vi "APT Control.vi"() -> ()   [LabVIEW 2015]
panel:
  in  "MG17Motor 5":refnum<k7>(container)
  in  "MG17Motor 4":refnum<k7>(container)
  in  "MG17Motor 3":refnum<k7>(container)
  in  "MG17Motor 2":refnum<k7>(container)
  in  "选项卡控件":enum32{"APT Controller", "Parameters"}(tab)
  in  "STOP Device":bool
  in  "Absolute 5":dbl
  in  "Absolute 4":dbl=1.0
  in  "Absolute 3":dbl
  in  "Absolute 2":dbl
  in  "Absolute 1":dbl
  in  "Stop":bool=TRUE
  in  "Home 1":bool
  in  "Rel. Pos 1":dbl=0.01 min=-10.0 max=360.0 format="%.2f"
  out "Display 1":dbl(knob) scale=0.0..50.0
  out "Initial 1":bool=TRUE
  in  "HWSerialNum 1":i32=90868400
  in  "1 Down":bool
  in  "1 Up":bool
  in  "HWSerialNum 2":i32=90868399
  out "Initial 2":bool=TRUE
  out "Display 2":dbl(knob) scale=0.0..25.0
  in  "2 Up":bool
  in  "2 Down":bool
  in  "HWSerialNum 3":i32=90843970
  out "Initial 3":bool=TRUE
  out "Display 3":dbl(knob)=0.9999828934669495 scale=0.0..25.0
  in  "3 Up":bool
  in  "3 Down":bool
  in  "Rel. Pos 3":dbl=0.01 min=-10.0 max=360.0 format="%.2f"
  in  "HWSerialNum 4":i32=90843969
  out "Initial 4":bool=TRUE
  out "Display 4":dbl(knob)=1.0 scale=0.0..50.0
  in  "4 Up":bool
  in  "4 Down":bool
  in  "Rel. Pos 4":dbl=0.1 min=-10.0 max=360.0 format="%.2f"
  in  "HWSerialNum 5":i32=90843968
  out "Initial 5":bool=TRUE
  out "Display 5":dbl(knob)=1.7000000476837158 scale=0.0..50.0
  in  "5 Up":bool
  in  "5 Down":bool
  in  "Rel. Pos 5":dbl=1.0 min=-10.0 max=360.0 format="%.2f"
  in  "Home 2":bool
  in  "Home 3":bool
  in  "Home 4":bool
  in  "Home 5":bool
  in  "Rel. Pos 2":dbl=0.01 min=-10.0 max=360.0 format="%.2f"
  in  "MG17Motor 1":refnum<k7>(container)
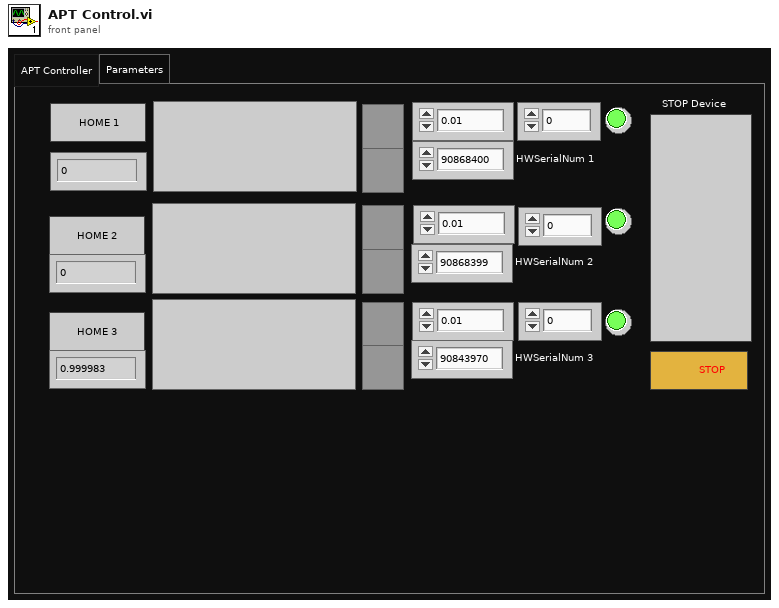
[diagram p1: front panel]
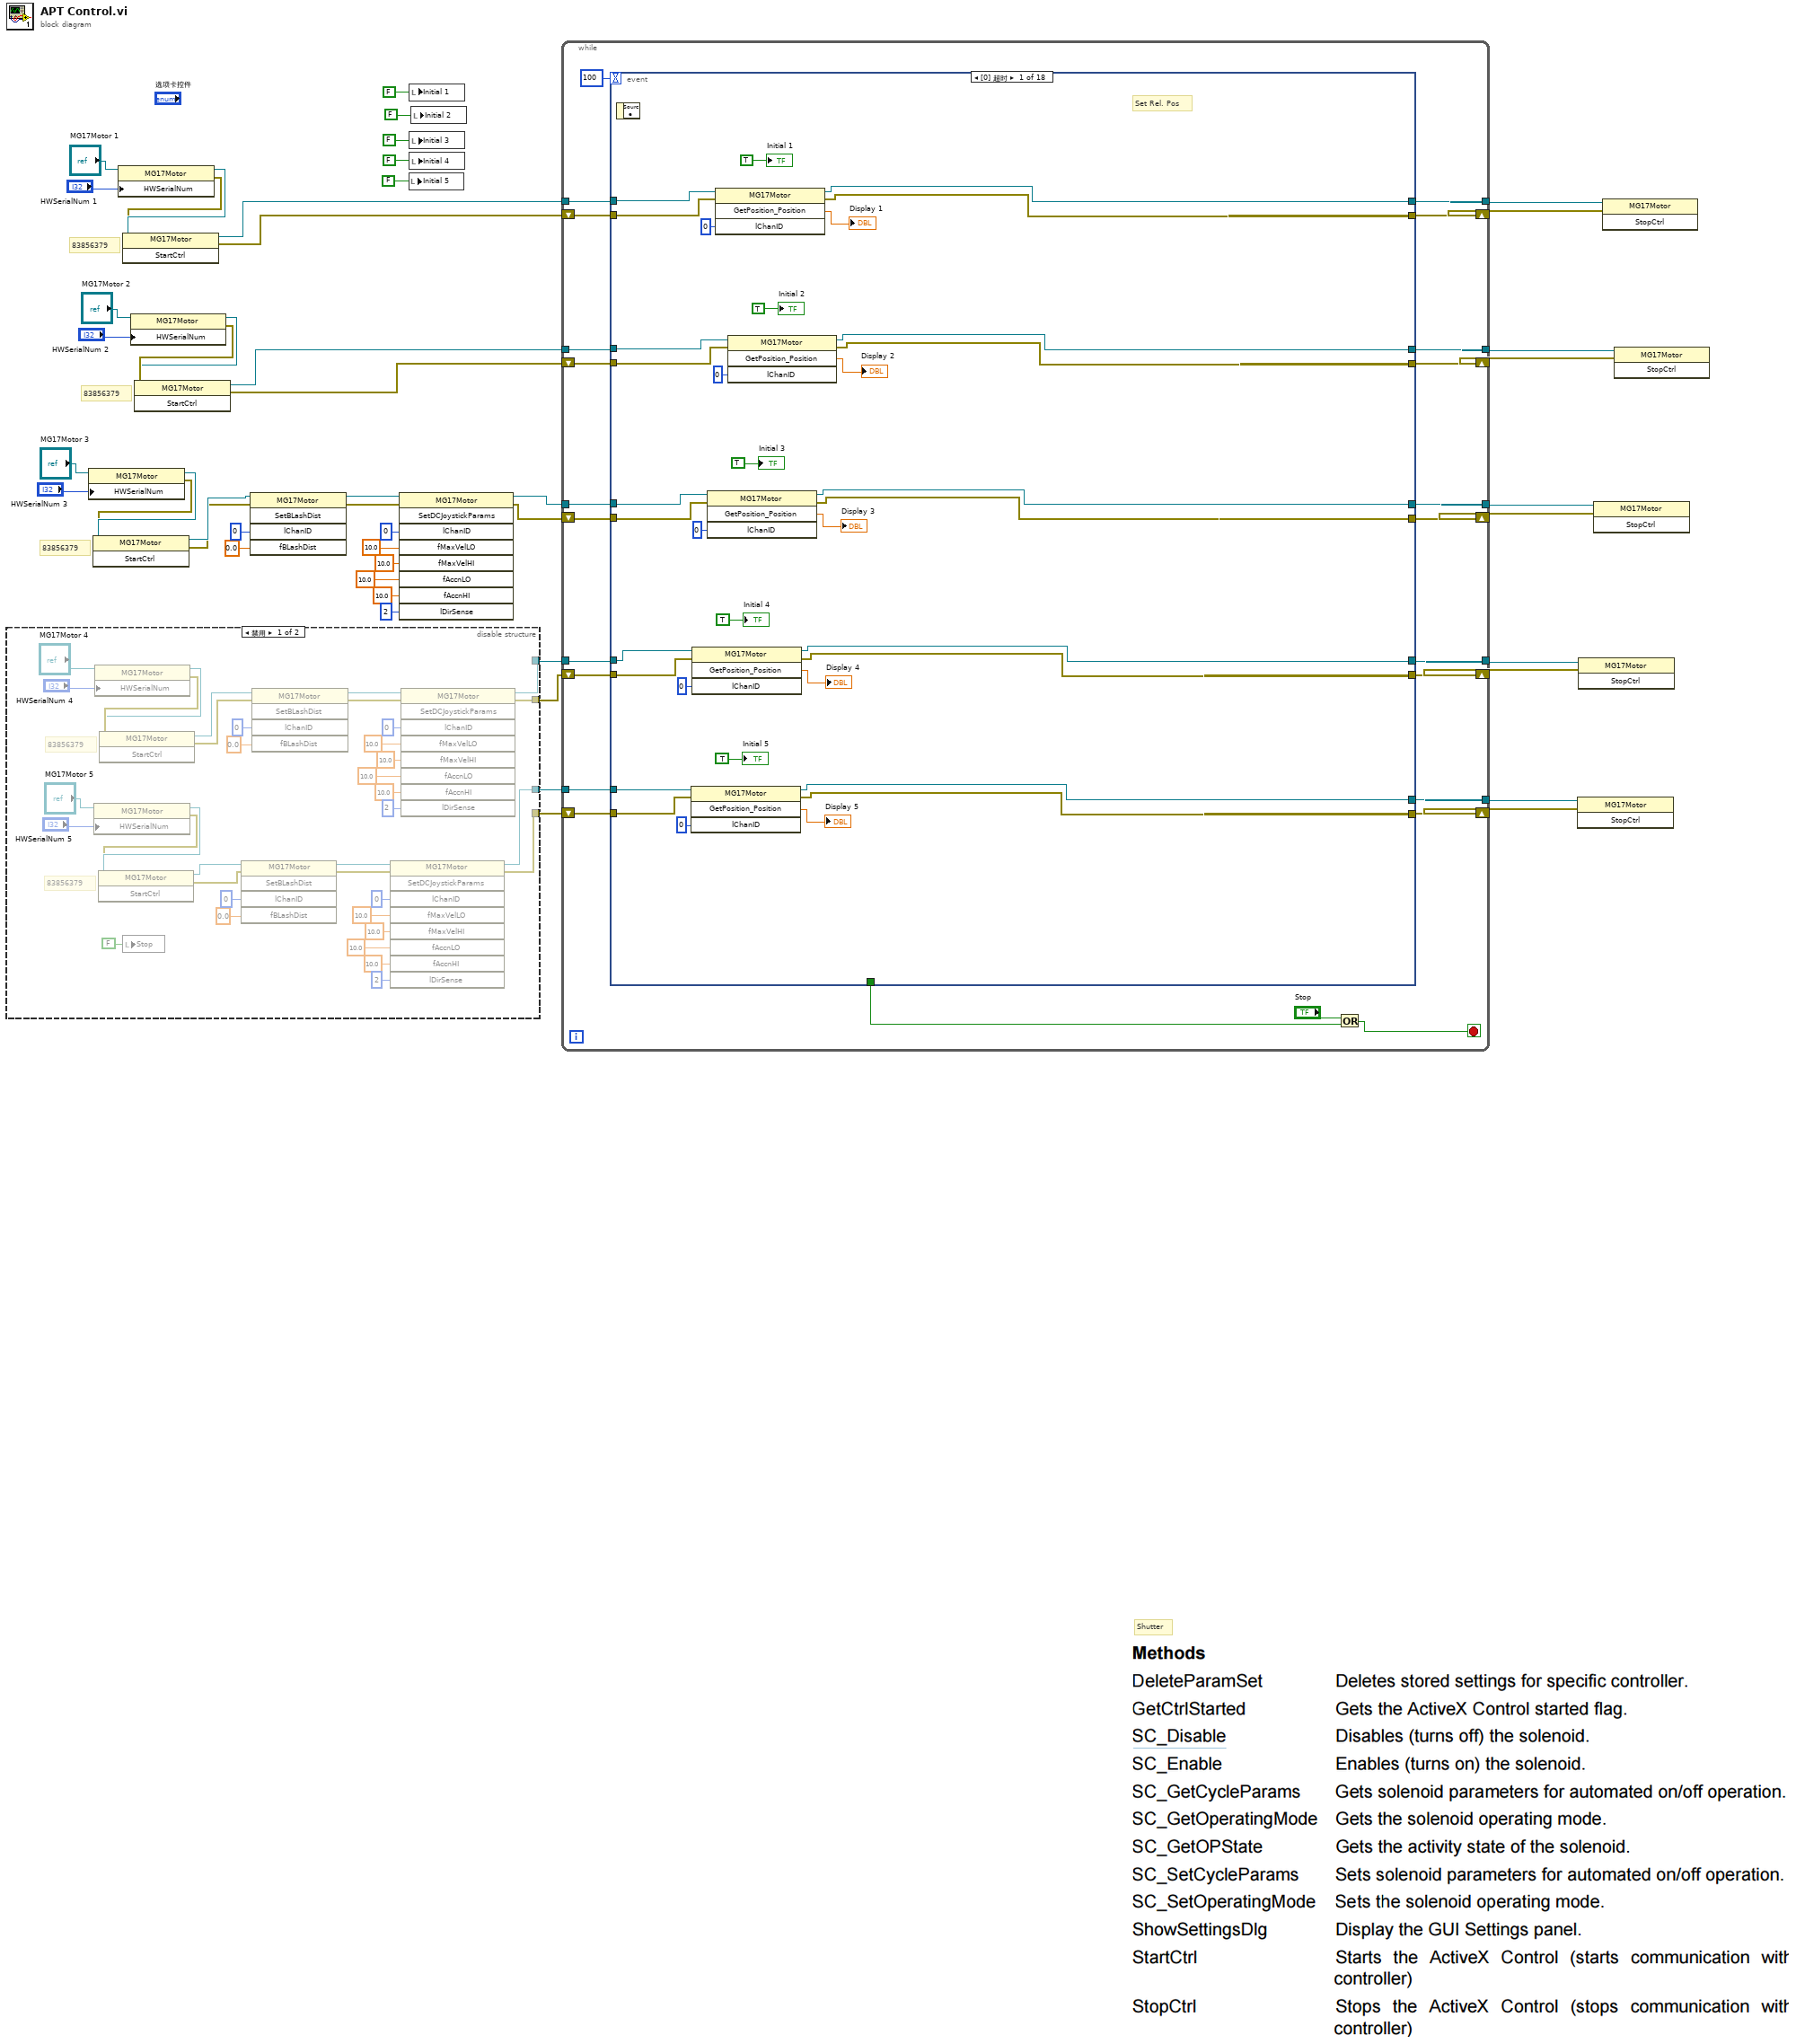
[diagram p0: block diagram]
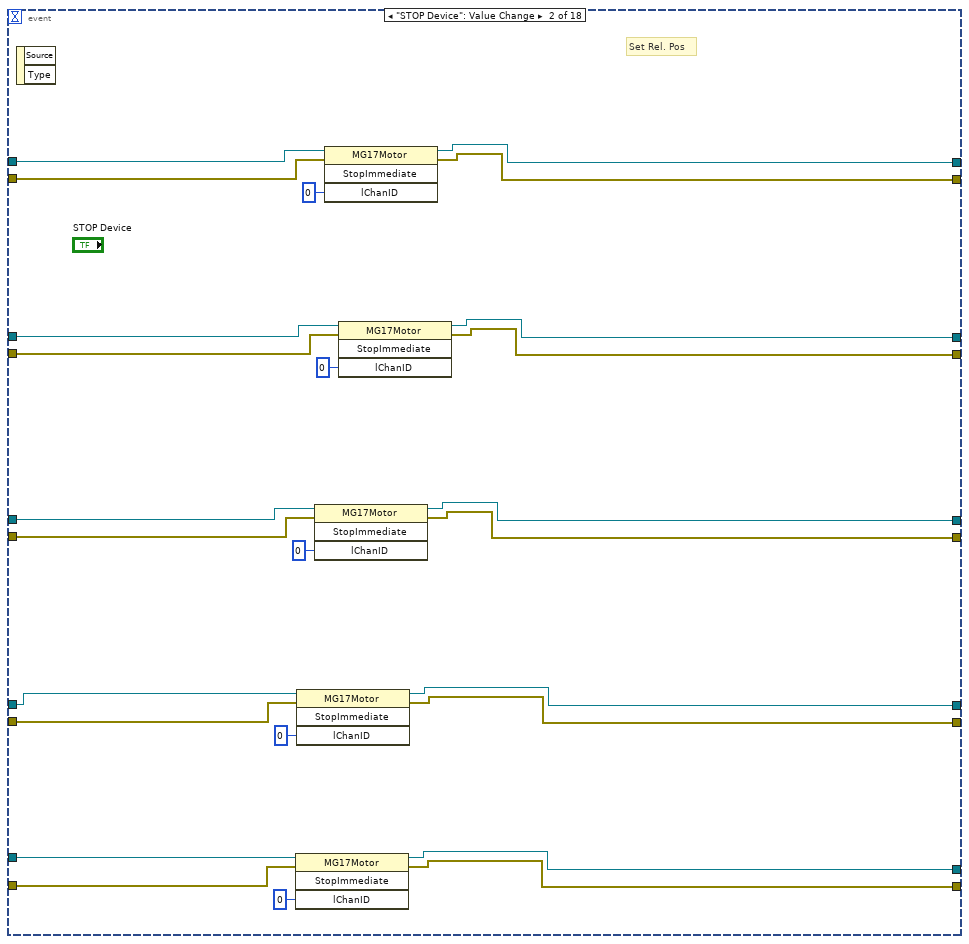
[diagram p3: hidden frame]
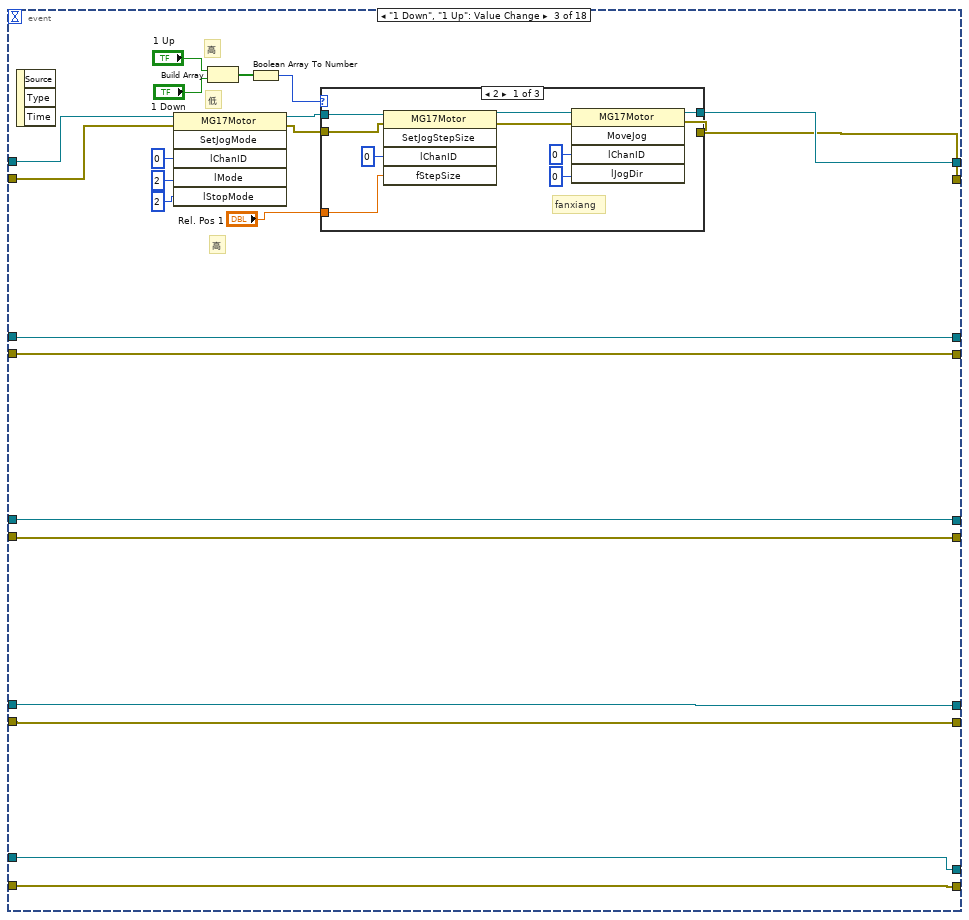
[diagram p4: hidden frame]
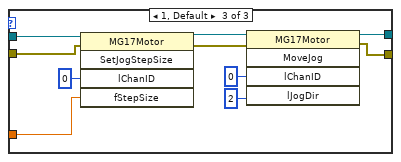
[diagram p6: hidden frame]
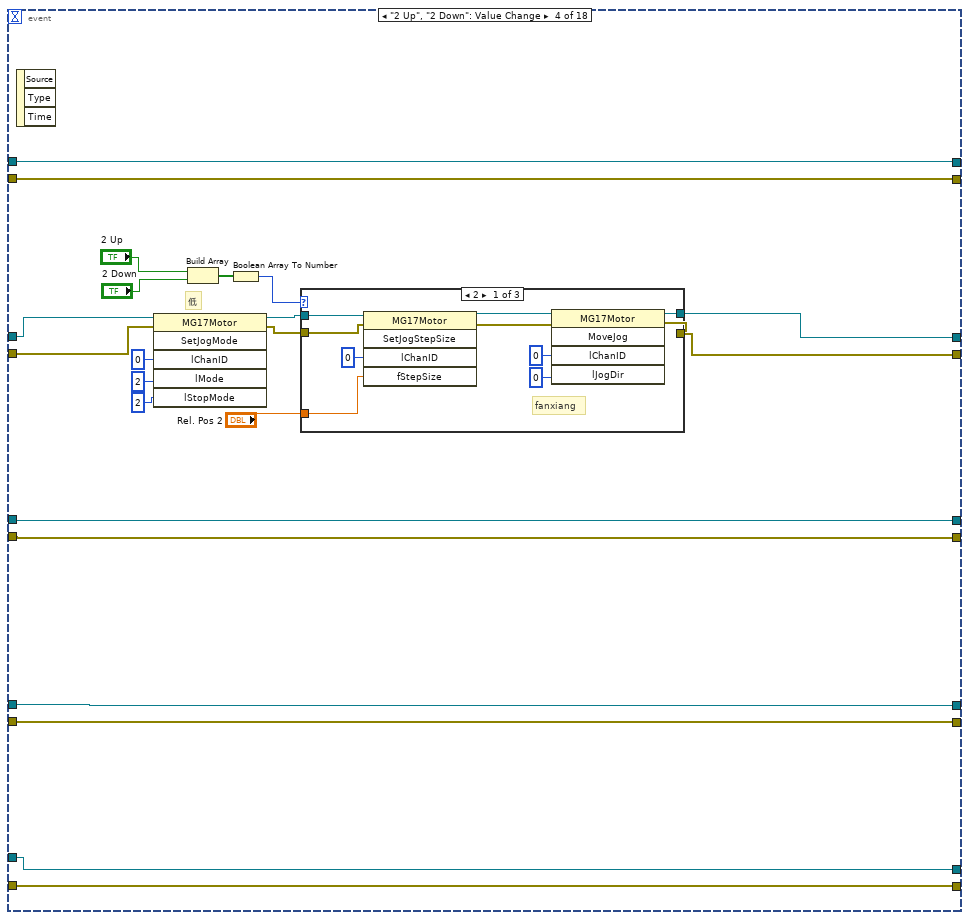
[diagram p7: hidden frame]
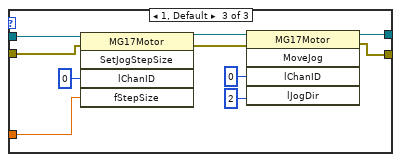
[diagram p9: hidden frame]
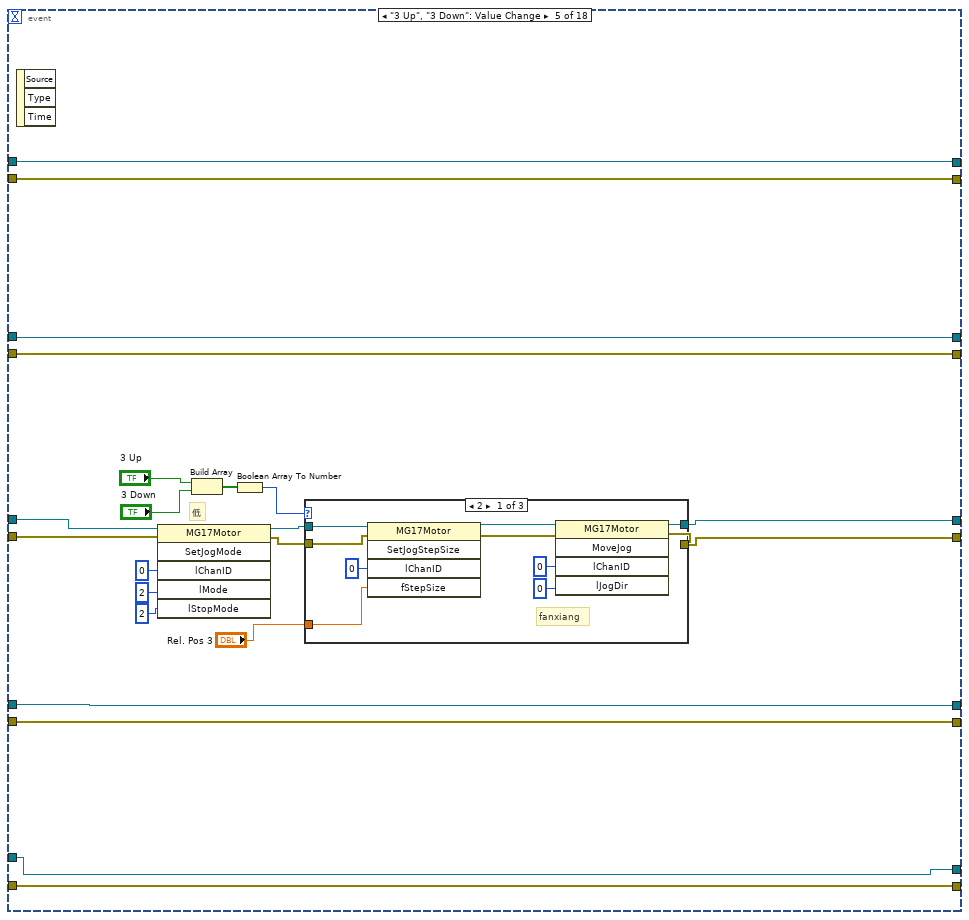
[diagram p10: hidden frame]
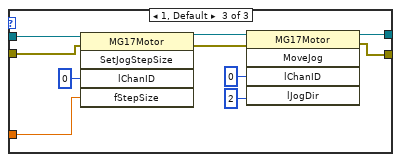
[diagram p12: hidden frame]
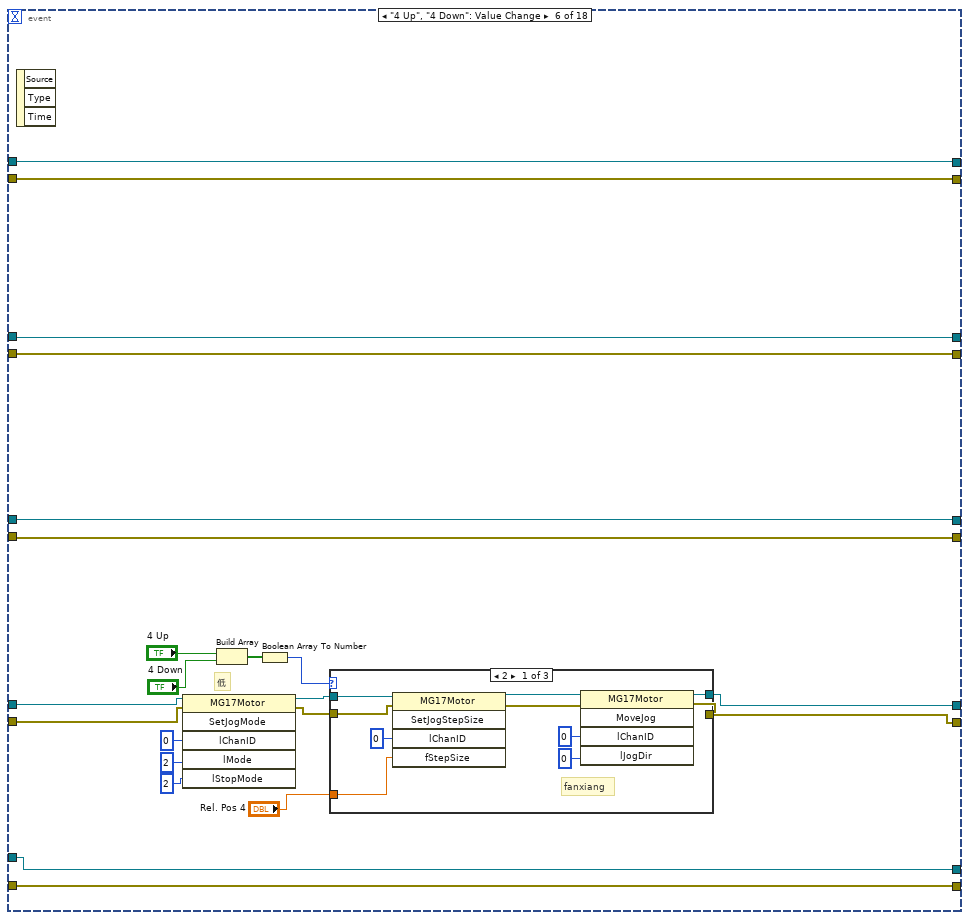
[diagram p13: hidden frame]
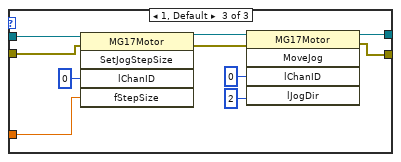
[diagram p15: hidden frame]
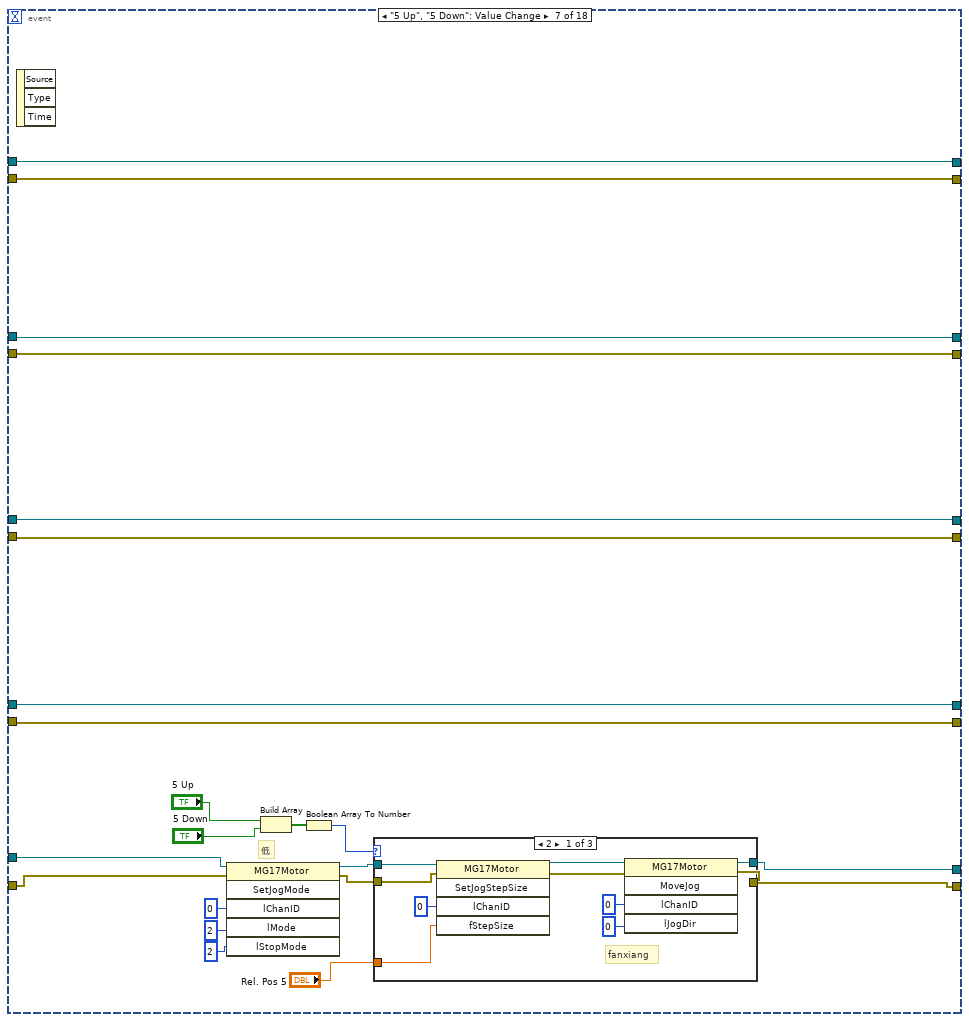
[diagram p16: hidden frame]
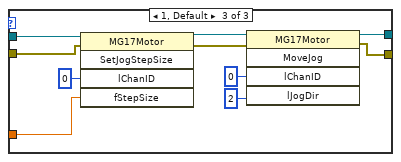
[diagram p18: hidden frame]
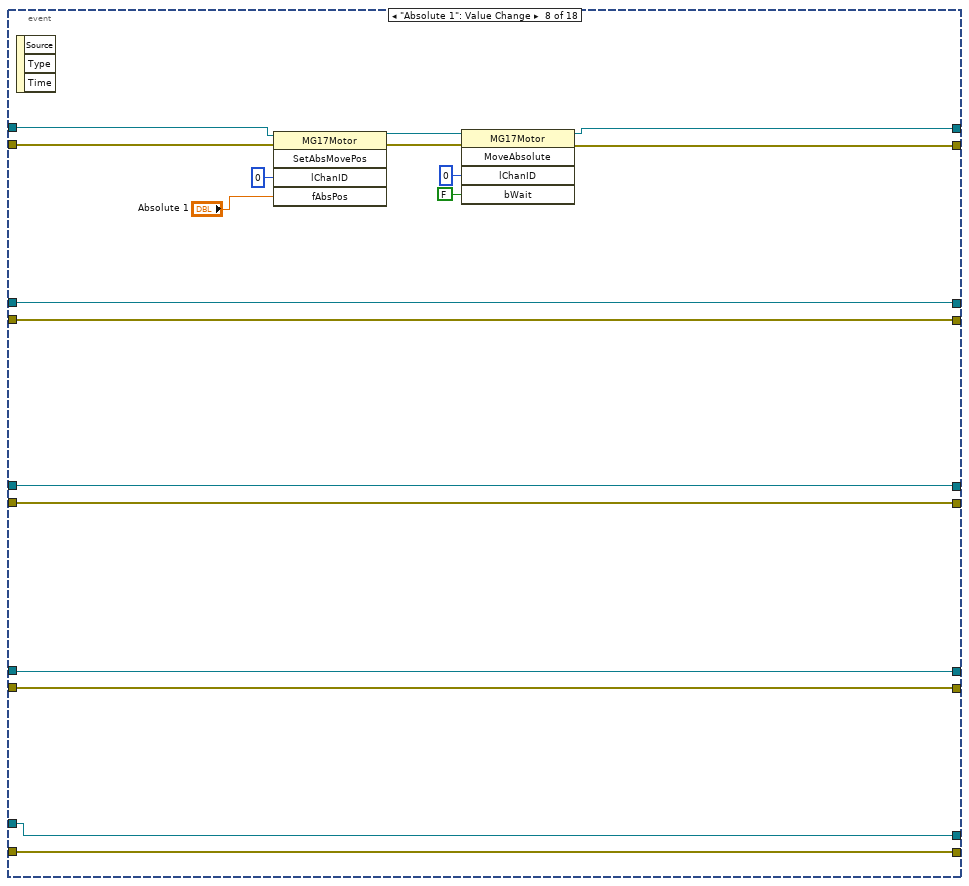
[diagram p19: hidden frame]
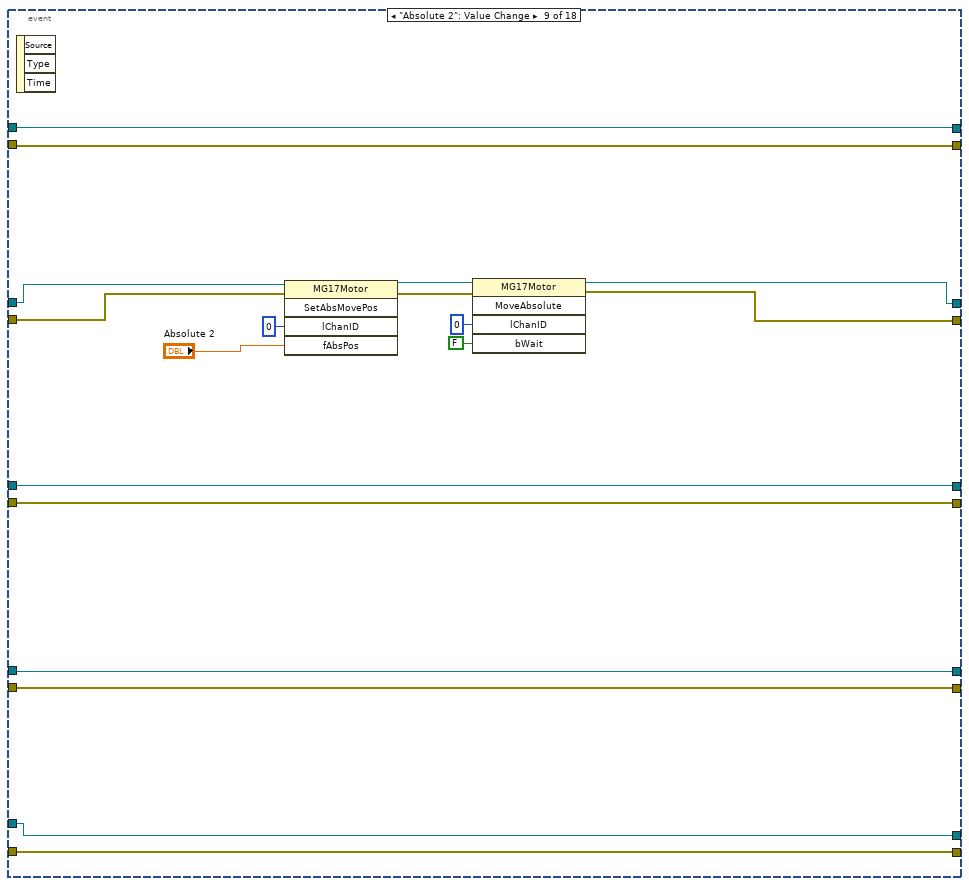
[diagram p20: hidden frame]
diagram:
  # "83856379"
  # "83856379"
  # "83856379"
  # "Shutter"
  n1 = disable-structure shown="禁用" {
    disable-tunnel: [w57 _] -> w18
    disable-tunnel: [w56 _] -> w17
    disable-tunnel: [w55 _] -> w16
    disable-tunnel: [w54 _] -> w15
    frame Disabled {
      # "83856379"
      # "83856379"
      n2 = property class="MG17Motor"(reference="MG17Motor 5", "HWSerialNum"="HWSerialNum 5") -> (reference out=w81:refnum<k7>, error out=w80:errorcluster)  [unwired: 1 in]
      n3 = property class="MG17Motor"(reference="MG17Motor 4", "HWSerialNum"="HWSerialNum 4") -> (reference out=w84:refnum<k7>, error out=w85:errorcluster)  [unwired: 1 in]
      n4 = invoke class="MG17Motor" method="StartCtrl"(reference=w81, error in=w80) -> (reference out=w53:refnum<k7>, error out=w52:errorcluster)  [unwired: 1 in, 1 out]
      n5 = invoke class="MG17Motor" method="StartCtrl"(reference=w84, error in=w85) -> (reference out=w51:refnum<k7>, error out=w50:errorcluster)  [unwired: 1 in, 1 out]
      n6 = local write "Stop"(FALSE ("Stop")) -> ()
      n7 = invoke class="MG17Motor" method="SetBLashDist"(reference=w53, error in=w52, "lChanID"=0, "fBLashDist"=sgl 0.0) -> (reference out=w75:refnum<k7>, error out=w74:errorcluster)  [unwired: 1 in, 3 out]
      n8 = invoke class="MG17Motor" method="SetBLashDist"(reference=w51, error in=w50, "lChanID"=0, "fBLashDist"=sgl 0.0) -> (reference out=w60:refnum<k7>, error out=w61:errorcluster)  [unwired: 1 in, 3 out]
      n9 = invoke class="MG17Motor" method="SetDCJoystickParams"(reference=w75, error in=w74, "lChanID"=0, "fMaxVelLO"=sgl 10.0, "fMaxVelHI"=sgl 10.0, "fAccnLO"=sgl 10.0, "fAccnHI"=sgl 10.0, "lDirSense"=2) -> (reference out=w55:refnum<k7>, error out=w54:errorcluster)  [unwired: 1 in, 7 out]
      n10 = invoke class="MG17Motor" method="SetDCJoystickParams"(reference=w60, error in=w61, "lChanID"=0, "fMaxVelLO"=sgl 10.0, "fMaxVelHI"=sgl 10.0, "fAccnLO"=sgl 10.0, "fAccnHI"=sgl 10.0, "lDirSense"=2) -> (reference out=w57:refnum<k7>, error out=w56:errorcluster)  [unwired: 1 in, 7 out]
    }
    frame Enabled {
    }
  }
  n11 = property class="MG17Motor"(reference="MG17Motor 3", "HWSerialNum"="HWSerialNum 3") -> (reference out=w31:refnum<k7>, error out=w30:errorcluster)  [unwired: 1 in]
  n12 = invoke class="MG17Motor" method="StartCtrl"(reference=w31, error in=w30) -> (reference out=w2:refnum<k7>, error out=w1:errorcluster)  [unwired: 1 in, 1 out]
  n13 = property class="MG17Motor"(reference="MG17Motor 1", "HWSerialNum"="HWSerialNum 1") -> (reference out=w48:refnum<k7>, error out=w47:errorcluster)  [unwired: 1 in]
  n14 = invoke class="MG17Motor" method="StartCtrl"(reference=w48, error in=w47) -> (reference out=w46:refnum<k7>, error out=w45:errorcluster)  [unwired: 1 in, 1 out]
  n15 = property class="MG17Motor"(reference="MG17Motor 2", "HWSerialNum"="HWSerialNum 2") -> (reference out=w34:refnum<k7>, error out=w35:errorcluster)  [unwired: 1 in]
  n16 = invoke class="MG17Motor" method="StartCtrl"(reference=w34, error in=w35) -> (reference out=w36:refnum<k7>, error out=w37:errorcluster)  [unwired: 1 in, 1 out]
  n17 = invoke class="MG17Motor" method="SetBLashDist"(reference=w2, error in=w1, "lChanID"=0, "fBLashDist"=sgl 0.0) -> (reference out=w12:refnum<k7>, error out=w11:errorcluster)  [unwired: 1 in, 3 out]
  n18 = invoke class="MG17Motor" method="SetDCJoystickParams"(reference=w12, error in=w11, "lChanID"=0, "fMaxVelLO"=sgl 10.0, "fMaxVelHI"=sgl 10.0, "fAccnLO"=sgl 10.0, "fAccnHI"=sgl 10.0, "lDirSense"=2) -> (reference out=w4:refnum<k7>, error out=w3:errorcluster)  [unwired: 1 in, 7 out]
  n19 = local write "Initial 5"(FALSE ("Initial")) -> ()
  n20 = local write "Initial 1"(FALSE ("Initial")) -> ()
  n21 = local write "Initial 3"(FALSE ("Initial")) -> ()
  n22 = local write "Initial 4"(FALSE ("Initial")) -> ()
  n23 = local write "Initial 2"(FALSE ("Initial")) -> ()
  n24 = while {
    shift-right: [w107] -> w43
    shift-left: w45 -> [w109]
    tunnel: w46 -> [w110]
    tunnel: [w108] -> w44
    shift-right: [w105] -> w39
    shift-left: w37 -> [w103]
    tunnel: w36 -> [w102]
    tunnel: [w104] -> w38
    shift-right: [w98] -> w28
    shift-left: w3 -> [w100]
    tunnel: w4 -> [w101]
    tunnel: [w99] -> w29
    shift-right: [w97] -> w26
    shift-left: w17 -> [w95]
    tunnel: w18 -> [w94]
    tunnel: [w96] -> w25
    shift-right: [w91] -> w23
    shift-left: w15 -> [w93]
    tunnel: [w92] -> w24
    tunnel: w16 -> [w87]
    stop <- w89 stop-if-true
    n25 = event shown="[0] 超时" {
      selector: _ -> [_ _ _ _ _ _ _ _ _ _ _ _ _ _ _ _ _ _]
      dyn-events: _ -> [_ _ _ _ _ _ _ _ _ _ _ _ _ _ _ _ _ _]
      timeout: 100 -> [_ _ _ _ _ _ _ _ _ _ _ _ _ _ _ _ _ _]
      tunnel: w110 -> [w144 w170 w183 w225 w273 w317 w361 w404 w411 w436 w456 w475 w491 w497 w514 w530 w545 w557]
      tunnel: w109 -> [w143 w169 w182 w224 w272 w316 w360 w403 w410 w435 w455 w474 w490 w496 w513 w529 w544 w556]
      tunnel: [w141 w168 w181 w225 w273 w317 w361 w394 w411 w436 w456 w475 w489 w497 w514 w530 w545 w557] -> w108
      tunnel: [w140 w167 w180 w224 w272 w316 w360 w393 w410 w435 w455 w474 w488 w496 w513 w529 w544 w556] -> w107
      tunnel: [_ _ _ _ _ _ _ _ _ _ _ _ _ _ _ _ _ TRUE ("Stop")] -> w88
      tunnel: w102 -> [w133 w163 w178 w229 w261 w314 w359 w402 w416 w429 w454 w473 w482 w499 w508 w528 w543 w555]
      tunnel: w103 -> [w134 w164 w177 w228 w260 w313 w358 w401 w415 w428 w453 w472 w481 w498 w507 w527 w542 w554]
      tunnel: [w136 w165 w178 w227 w261 w314 w359 w402 w414 w429 w454 w473 w482 w495 w508 w528 w543 w555] -> w104
      tunnel: [w137 w166 w177 w226 w260 w313 w358 w401 w413 w428 w453 w472 w481 w494 w507 w527 w542 w554] -> w105
      tunnel: w101 -> [w130 w162 w176 w220 w265 w306 w357 w400 w422 w433 w447 w471 w484 w501 w512 w522 w541 w553]
      tunnel: w100 -> [w129 w161 w175 w219 w264 w305 w356 w399 w421 w430 w446 w470 w483 w500 w511 w521 w540 w552]
      tunnel: [w127 w160 w176 w220 w263 w306 w357 w400 w422 w432 w447 w471 w484 w501 w510 w522 w541 w553] -> w99
      tunnel: [w126 w159 w175 w219 w262 w305 w356 w399 w421 w431 w446 w470 w483 w500 w509 w521 w540 w552] -> w98
      tunnel: w94 -> [w119 w155 w174 w218 w271 w310 w349 w398 w420 w440 w451 w465 w486 w503 w516 w526 w536 w551]
      tunnel: w95 -> [w120 w156 w173 w217 w270 w309 w348 w397 w419 w439 w450 w464 w485 w502 w515 w525 w535 w550]
      tunnel: [w122 w157 w174 w218 w271 w308 w349 w398 w420 w440 w449 w465 w486 w503 w516 w524 w536 w551] -> w96
      tunnel: [w123 w158 w173 w217 w270 w307 w348 w397 w419 w439 w448 w464 w485 w502 w515 w523 w535 w550] -> w97
      tunnel: w93 -> [w116 w154 w172 w216 w269 w315 w355 w396 w418 w438 w458 w468 w487 w504 w517 w531 w539 w549]
      tunnel: [w114 w153 w171 w215 w259 w303 w354 w391 w409 w427 w445 w467 _ _ _ w520 w538 w548] -> w92
      tunnel: [w113 w152 w172 w216 w269 w315 w353 w396 w418 w438 w458 w466 w487 w504 w517 w531 w537 w549] -> w91
      tunnel: w87 -> [w111 w151 w171 w215 w259 w303 w347 w391 w409 w427 w445 w463 _ _ _ w520 w534 w548]
      event Timeout {
        # "Set Rel. Pos"
        n26 = event-data() -> ()  [unwired: 1 in, 1 out]
        n27 = invoke class="MG17Motor" method="GetPosition_Position"(reference=w111, error in=w116, "lChanID"=0) -> (reference out=w114:refnum<k7>, error out=w113:errorcluster, "GetPosition_Position"=→"Display 5":sgl)  [unwired: 1 in, 1 out]
        n28 = invoke class="MG17Motor" method="GetPosition_Position"(reference=w119, error in=w120, "lChanID"=0) -> (reference out=w122:refnum<k7>, error out=w123:errorcluster, "GetPosition_Position"=→"Display 4":sgl)  [unwired: 1 in, 1 out]
        n29 = invoke class="MG17Motor" method="GetPosition_Position"(reference=w130, error in=w129, "lChanID"=0) -> (reference out=w127:refnum<k7>, error out=w126:errorcluster, "GetPosition_Position"=→"Display 3":sgl)  [unwired: 1 in, 1 out]
        n30 = invoke class="MG17Motor" method="GetPosition_Position"(reference=w144, error in=w143, "lChanID"=0) -> (reference out=w141:refnum<k7>, error out=w140:errorcluster, "GetPosition_Position"=→"Display 1":sgl)  [unwired: 1 in, 1 out]
        n31 = invoke class="MG17Motor" method="GetPosition_Position"(reference=w133, error in=w134, "lChanID"=0) -> (reference out=w136:refnum<k7>, error out=w137:errorcluster, "GetPosition_Position"=→"Display 2":sgl)  [unwired: 1 in, 1 out]
        "Initial 1" <- TRUE ("Initial")
        "Initial 2" <- TRUE ("Initial")
        "Initial 3" <- TRUE ("Initial")
        "Initial 4" <- TRUE ("Initial")
        "Initial 5" <- TRUE ("Initial")
      }
      event "STOP Device": Value Change {
        # "Set Rel. Pos"
        n32 = event-data() -> ()  [unwired: 1 in, 2 out]
        n33 = invoke class="MG17Motor" method="StopImmediate"(reference=w151, error in=w154, "lChanID"=0) -> (reference out=w153:refnum<k7>, error out=w152:errorcluster)  [unwired: 1 in, 2 out]
        n34 = invoke class="MG17Motor" method="StopImmediate"(reference=w155, error in=w156, "lChanID"=0) -> (reference out=w157:refnum<k7>, error out=w158:errorcluster)  [unwired: 1 in, 2 out]
        n35 = invoke class="MG17Motor" method="StopImmediate"(reference=w162, error in=w161, "lChanID"=0) -> (reference out=w160:refnum<k7>, error out=w159:errorcluster)  [unwired: 1 in, 2 out]
        n36 = invoke class="MG17Motor" method="StopImmediate"(reference=w170, error in=w169, "lChanID"=0) -> (reference out=w168:refnum<k7>, error out=w167:errorcluster)  [unwired: 1 in, 2 out]
        n37 = invoke class="MG17Motor" method="StopImmediate"(reference=w163, error in=w164, "lChanID"=0) -> (reference out=w165:refnum<k7>, error out=w166:errorcluster)  [unwired: 1 in, 2 out]
      }
      event "1 Down", "1 Up": Value Change {
        # "高"
        # "低"
        # "高"
        n38 = event-data() -> ()  [unwired: 1 in, 3 out]
        n39 = invoke class="MG17Motor" method="SetJogMode"(reference=w183, error in=w182, "lChanID"=0, "lMode"=2, "lStopMode"=2) -> (reference out=w188:refnum<k7>, error out=w189:errorcluster)  [unwired: 1 in, 4 out]
        n40 = Build Array("1 Up", "1 Down") -> (w186:bool[])
        n41 = Boolean Array To Number(Boolean array=w186) -> (number=w187:u32)
        n42 = case shown="2" w187 {
          tunnel: w188 -> [w202 w204 w214]
          tunnel: [w200 w204 w212] -> w181
          tunnel: w189 -> [w197 w203 w209]
          tunnel: [w195 w203 w207] -> w180
          tunnel: "Rel. Pos 1" -> [w193 _ w205]
          frame 2 {
            # "fanxiang"
            n43 = invoke class="MG17Motor" method="SetJogStepSize"(reference=w202, error in=w197, "lChanID"=0, "fStepSize"=w193) -> (reference out=w201:refnum<k7>, error out=w196:errorcluster)  [unwired: 1 in, 3 out]
            n44 = invoke class="MG17Motor" method="MoveJog"(reference=w201, error in=w196, "lChanID"=0, "lJogDir"=0) -> (reference out=w200:refnum<k7>, error out=w195:errorcluster)  [unwired: 1 in, 3 out]
          }
          frame 0 {
          }
          frame 1, Default {
            n45 = invoke class="MG17Motor" method="SetJogStepSize"(reference=w214, error in=w209, "lChanID"=0, "fStepSize"=w205) -> (reference out=w213:refnum<k7>, error out=w208:errorcluster)  [unwired: 1 in, 3 out]
            n46 = invoke class="MG17Motor" method="MoveJog"(reference=w213, error in=w208, "lChanID"=0, "lJogDir"=2) -> (reference out=w212:refnum<k7>, error out=w207:errorcluster)  [unwired: 1 in, 3 out]
          }
        }
      }
      event "2 Up", "2 Down": Value Change {
        # "低"
        n47 = event-data() -> ()  [unwired: 1 in, 3 out]
        n48 = invoke class="MG17Motor" method="SetJogMode"(reference=w229, error in=w228, "lChanID"=0, "lMode"=2, "lStopMode"=2) -> (reference out=w234:refnum<k7>, error out=w233:errorcluster)  [unwired: 1 in, 4 out]
        n49 = Build Array("2 Up", "2 Down") -> (w236:bool[])
        n50 = Boolean Array To Number(Boolean array=w236) -> (number=w235:u32)
        n51 = case shown="2" w235 {
          tunnel: w234 -> [w246 w248 w258]
          tunnel: [w244 w248 w256] -> w227
          tunnel: w233 -> [w241 w247 w253]
          tunnel: [w239 w247 w251] -> w226
          tunnel: "Rel. Pos 2" -> [w237 _ w249]
          frame 2 {
            # "fanxiang"
            n52 = invoke class="MG17Motor" method="SetJogStepSize"(reference=w246, error in=w241, "lChanID"=0, "fStepSize"=w237) -> (reference out=w245:refnum<k7>, error out=w240:errorcluster)  [unwired: 1 in, 3 out]
            n53 = invoke class="MG17Motor" method="MoveJog"(reference=w245, error in=w240, "lChanID"=0, "lJogDir"=0) -> (reference out=w244:refnum<k7>, error out=w239:errorcluster)  [unwired: 1 in, 3 out]
          }
          frame 0 {
          }
          frame 1, Default {
            n54 = invoke class="MG17Motor" method="SetJogStepSize"(reference=w258, error in=w253, "lChanID"=0, "fStepSize"=w249) -> (reference out=w257:refnum<k7>, error out=w252:errorcluster)  [unwired: 1 in, 3 out]
            n55 = invoke class="MG17Motor" method="MoveJog"(reference=w257, error in=w252, "lChanID"=0, "lJogDir"=2) -> (reference out=w256:refnum<k7>, error out=w251:errorcluster)  [unwired: 1 in, 3 out]
          }
        }
      }
      event "3 Up", "3 Down": Value Change {
        # "低"
        n56 = event-data() -> ()  [unwired: 1 in, 3 out]
        n57 = invoke class="MG17Motor" method="SetJogMode"(reference=w265, error in=w264, "lChanID"=0, "lMode"=2, "lStopMode"=2) -> (reference out=w278:refnum<k7>, error out=w277:errorcluster)  [unwired: 1 in, 4 out]
        n58 = Build Array("3 Up", "3 Down") -> (w280:bool[])
        n59 = Boolean Array To Number(Boolean array=w280) -> (number=w279:u32)
        n60 = case shown="2" w279 {
          tunnel: w278 -> [w290 w292 w302]
          tunnel: [w288 w292 w300] -> w263
          tunnel: w277 -> [w285 w291 w297]
          tunnel: [w283 w291 w295] -> w262
          tunnel: "Rel. Pos 3" -> [w281 _ w293]
          frame 2 {
            # "fanxiang"
            n61 = invoke class="MG17Motor" method="SetJogStepSize"(reference=w290, error in=w285, "lChanID"=0, "fStepSize"=w281) -> (reference out=w289:refnum<k7>, error out=w284:errorcluster)  [unwired: 1 in, 3 out]
            n62 = invoke class="MG17Motor" method="MoveJog"(reference=w289, error in=w284, "lChanID"=0, "lJogDir"=0) -> (reference out=w288:refnum<k7>, error out=w283:errorcluster)  [unwired: 1 in, 3 out]
          }
          frame 0 {
          }
          frame 1, Default {
            n63 = invoke class="MG17Motor" method="SetJogStepSize"(reference=w302, error in=w297, "lChanID"=0, "fStepSize"=w293) -> (reference out=w301:refnum<k7>, error out=w296:errorcluster)  [unwired: 1 in, 3 out]
            n64 = invoke class="MG17Motor" method="MoveJog"(reference=w301, error in=w296, "lChanID"=0, "lJogDir"=2) -> (reference out=w300:refnum<k7>, error out=w295:errorcluster)  [unwired: 1 in, 3 out]
          }
        }
      }
      event "4 Up", "4 Down": Value Change {
        # "低"
        n65 = event-data() -> ()  [unwired: 1 in, 3 out]
        n66 = invoke class="MG17Motor" method="SetJogMode"(reference=w310, error in=w309, "lChanID"=0, "lMode"=2, "lStopMode"=2) -> (reference out=w322:refnum<k7>, error out=w321:errorcluster)  [unwired: 1 in, 4 out]
        n67 = Build Array("4 Up", "4 Down") -> (w324:bool[])
        n68 = Boolean Array To Number(Boolean array=w324) -> (number=w323:u32)
        n69 = case shown="2" w323 {
          tunnel: w322 -> [w334 w336 w346]
          tunnel: [w332 w336 w344] -> w308
          tunnel: w321 -> [w329 w335 w341]
          tunnel: [w327 w335 w339] -> w307
          tunnel: "Rel. Pos 4" -> [w325 _ w337]
          frame 2 {
            # "fanxiang"
            n70 = invoke class="MG17Motor" method="SetJogStepSize"(reference=w334, error in=w329, "lChanID"=0, "fStepSize"=w325) -> (reference out=w333:refnum<k7>, error out=w328:errorcluster)  [unwired: 1 in, 3 out]
            n71 = invoke class="MG17Motor" method="MoveJog"(reference=w333, error in=w328, "lChanID"=0, "lJogDir"=0) -> (reference out=w332:refnum<k7>, error out=w327:errorcluster)  [unwired: 1 in, 3 out]
          }
          frame 0 {
          }
          frame 1, Default {
            n72 = invoke class="MG17Motor" method="SetJogStepSize"(reference=w346, error in=w341, "lChanID"=0, "fStepSize"=w337) -> (reference out=w345:refnum<k7>, error out=w340:errorcluster)  [unwired: 1 in, 3 out]
            n73 = invoke class="MG17Motor" method="MoveJog"(reference=w345, error in=w340, "lChanID"=0, "lJogDir"=2) -> (reference out=w344:refnum<k7>, error out=w339:errorcluster)  [unwired: 1 in, 3 out]
          }
        }
      }
      event "5 Up", "5 Down": Value Change {
        # "低"
        n74 = event-data() -> ()  [unwired: 1 in, 3 out]
        n75 = invoke class="MG17Motor" method="SetJogMode"(reference=w347, error in=w355, "lChanID"=0, "lMode"=2, "lStopMode"=2) -> (reference out=w366:refnum<k7>, error out=w365:errorcluster)  [unwired: 1 in, 4 out]
        n76 = Build Array("5 Up", "5 Down") -> (w368:bool[])
        n77 = Boolean Array To Number(Boolean array=w368) -> (number=w367:u32)
        n78 = case shown="2" w367 {
          tunnel: w366 -> [w378 w380 w390]
          tunnel: [w376 w380 w388] -> w354
          tunnel: w365 -> [w373 w379 w385]
          tunnel: [w371 w379 w383] -> w353
          tunnel: "Rel. Pos 5" -> [w369 _ w381]
          frame 2 {
            # "fanxiang"
            n79 = invoke class="MG17Motor" method="SetJogStepSize"(reference=w378, error in=w373, "lChanID"=0, "fStepSize"=w369) -> (reference out=w377:refnum<k7>, error out=w372:errorcluster)  [unwired: 1 in, 3 out]
            n80 = invoke class="MG17Motor" method="MoveJog"(reference=w377, error in=w372, "lChanID"=0, "lJogDir"=0) -> (reference out=w376:refnum<k7>, error out=w371:errorcluster)  [unwired: 1 in, 3 out]
          }
          frame 0 {
          }
          frame 1, Default {
            n81 = invoke class="MG17Motor" method="SetJogStepSize"(reference=w390, error in=w385, "lChanID"=0, "fStepSize"=w381) -> (reference out=w389:refnum<k7>, error out=w384:errorcluster)  [unwired: 1 in, 3 out]
            n82 = invoke class="MG17Motor" method="MoveJog"(reference=w389, error in=w384, "lChanID"=0, "lJogDir"=2) -> (reference out=w388:refnum<k7>, error out=w383:errorcluster)  [unwired: 1 in, 3 out]
          }
        }
      }
      event "Absolute 1": Value Change {
        n83 = event-data() -> ()  [unwired: 1 in, 3 out]
        n84 = invoke class="MG17Motor" method="SetAbsMovePos"(reference=w404, error in=w403, "lChanID"=0, "fAbsPos"="Absolute 1") -> (reference out=w408:refnum<k7>, error out=w405:errorcluster)  [unwired: 1 in, 3 out]
        n85 = invoke class="MG17Motor" method="MoveAbsolute"(reference=w408, error in=w405, "lChanID"=0, "bWait"=FALSE) -> (reference out=w394:refnum<k7>, error out=w393:errorcluster)  [unwired: 1 in, 3 out]
      }
      event "Absolute 2": Value Change {
        n86 = event-data() -> ()  [unwired: 1 in, 3 out]
        n87 = invoke class="MG17Motor" method="SetAbsMovePos"(reference=w416, error in=w415, "lChanID"=0, "fAbsPos"="Absolute 2") -> (reference out=w426:refnum<k7>, error out=w423:errorcluster)  [unwired: 1 in, 3 out]
        n88 = invoke class="MG17Motor" method="MoveAbsolute"(reference=w426, error in=w423, "lChanID"=0, "bWait"=FALSE) -> (reference out=w414:refnum<k7>, error out=w413:errorcluster)  [unwired: 1 in, 3 out]
      }
      event "Absolute 3": Value Change {
        n89 = event-data() -> ()  [unwired: 1 in, 3 out]
        n90 = invoke class="MG17Motor" method="SetAbsMovePos"(reference=w433, error in=w430, "lChanID"=0, "fAbsPos"="Absolute 3") -> (reference out=w444:refnum<k7>, error out=w441:errorcluster)  [unwired: 1 in, 3 out]
        n91 = invoke class="MG17Motor" method="MoveAbsolute"(reference=w444, error in=w441, "lChanID"=0, "bWait"=FALSE) -> (reference out=w432:refnum<k7>, error out=w431:errorcluster)  [unwired: 1 in, 3 out]
      }
      event "Absolute 4": Value Change {
        n92 = event-data() -> ()  [unwired: 1 in, 3 out]
        n93 = invoke class="MG17Motor" method="SetAbsMovePos"(reference=w451, error in=w450, "lChanID"=0, "fAbsPos"="Absolute 4") -> (reference out=w462:refnum<k7>, error out=w459:errorcluster)  [unwired: 1 in, 3 out]
        n94 = invoke class="MG17Motor" method="MoveAbsolute"(reference=w462, error in=w459, "lChanID"=0, "bWait"=FALSE) -> (reference out=w449:refnum<k7>, error out=w448:errorcluster)  [unwired: 1 in, 3 out]
      }
      event "Absolute 5": Value Change {
        n95 = event-data() -> ()  [unwired: 1 in, 3 out]
        n96 = invoke class="MG17Motor" method="SetAbsMovePos"(reference=w463, error in=w468, "lChanID"=0, "fAbsPos"="Absolute 5") -> (reference out=w480:refnum<k7>, error out=w477:errorcluster)  [unwired: 1 in, 3 out]
        n97 = invoke class="MG17Motor" method="MoveAbsolute"(reference=w480, error in=w477, "lChanID"=0, "bWait"=FALSE) -> (reference out=w467:refnum<k7>, error out=w466:errorcluster)  [unwired: 1 in, 3 out]
      }
      event "Home 1": Value Change {
        # "Home"
        n98 = event-data() -> ()  [unwired: 1 in, 3 out]
        n99 = invoke class="MG17Motor" method="MoveHome"(reference=w491, error in=w490, "lChanID"=0, "bWait"=FALSE) -> (reference out=w489:refnum<k7>, error out=w488:errorcluster)  [unwired: 1 in, 3 out]
      }
      event "Home 2": Value Change {
        # "Home"
        n100 = event-data() -> ()  [unwired: 1 in, 3 out]
        n101 = invoke class="MG17Motor" method="MoveHome"(reference=w499, error in=w498, "lChanID"=0, "bWait"=FALSE) -> (reference out=w495:refnum<k7>, error out=w494:errorcluster)  [unwired: 1 in, 3 out]
      }
      event "Home 3": Value Change {
        # "Home"
        n102 = event-data() -> ()  [unwired: 1 in, 3 out]
        n103 = invoke class="MG17Motor" method="MoveHome"(reference=w512, error in=w511, "lChanID"=0, "bWait"=FALSE) -> (reference out=w510:refnum<k7>, error out=w509:errorcluster)  [unwired: 1 in, 3 out]
      }
      event "Home 4": Value Change {
        # "Home"
        n104 = event-data() -> ()  [unwired: 1 in, 3 out]
        n105 = invoke class="MG17Motor" method="MoveHome"(reference=w526, error in=w525, "lChanID"=0, "bWait"=FALSE) -> (reference out=w524:refnum<k7>, error out=w523:errorcluster)  [unwired: 1 in, 3 out]
      }
      event "Home 5": Value Change {
        # "Home"
        n106 = event-data() -> ()  [unwired: 1 in, 3 out]
        n107 = invoke class="MG17Motor" method="MoveHome"(reference=w534, error in=w539, "lChanID"=0, "bWait"=FALSE) -> (reference out=w538:refnum<k7>, error out=w537:errorcluster)  [unwired: 1 in, 3 out]
      }
      event "Stop": Value Change {
        n108 = event-data() -> ()  [unwired: 1 in, 2 out]
      }
    }
    n109 = Or(x="Stop", y=w88) -> (x .or. y?=w89:bool)
  }
  n110 = invoke class="MG17Motor" method="StopCtrl"(reference=w24, error in=w23) -> ()  [unwired: 1 in, 3 out]
  n111 = invoke class="MG17Motor" method="StopCtrl"(reference=w25, error in=w26) -> ()  [unwired: 1 in, 3 out]
  n112 = invoke class="MG17Motor" method="StopCtrl"(reference=w29, error in=w28) -> ()  [unwired: 1 in, 3 out]
  n113 = invoke class="MG17Motor" method="StopCtrl"(reference=w44, error in=w43) -> ()  [unwired: 1 in, 3 out]
  n114 = invoke class="MG17Motor" method="StopCtrl"(reference=w38, error in=w39) -> ()  [unwired: 1 in, 3 out]
